vi "Get Shooter RPM.vi"() -> (1 "Average RPM":dbl, 2 "Right RPM":dbl, 3 "Left RPM":dbl)   [LabVIEW 2015]
uses:
  Robot Global Data.vi
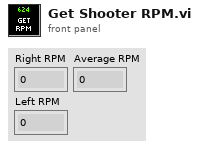
[diagram p1: front panel]
types:
  T1 = typedef "Dashboard Control Data.ctl" = cluster{"Auton Loops":dbl, "Shooter Presets":T2, "Encoder Control":T4, "Steer PID output":cluster{"output high":dbl, "output low":dbl}, " Steer PID gains":cluster{"proportional gain (Kc)":dbl, "integral time (Ti, min)":dbl, "derivative time (Td, min)":dbl}, "Drivetrain Settings":T5, "Vision Packet":T6, "Dashboard Drivetrain Command":T7}
  T2 = typedef "Shooter Presets.ctl" = cluster{"Batter Shot":T3, "Low Bar Curve Shot":T3, "Deep Middle Shot":T3, "Manual Shot":T3, "Left Ticks Per Rotation":dbl, "Right Ticks Per Rotation":dbl, "Low Bar Shot":T3, "Shooter RPM Tolerance":dbl, "IIR Filter Power":dbl}
  T3 = typedef "Shot Presets.ctl" = cluster{"Left Wheel RPM":dbl, "Right Wheel RPM":dbl}
  T4 = typedef "Encoder Control.ctl" = cluster{"Right Tick Constat":dbl, "Left Tick Constant":dbl, "Reset?":bool, "Y Dist":cluster{"PID gains":cluster{"proportional gain (Kc)":dbl, "integral time (Ti, min)":dbl, "derivative time (Td, min)":dbl}}, "Y Stop Thresh":dbl, "Y Stop Speed":dbl}
  T5 = typedef "Drivetrain Settings.ctl" = cluster{"Gyro Tolerance":dbl, "Throttle Ramp (ms)":dbl, "Angular rate compensation":bool, "Throttle to Rate Scale":dbl, "Rate compensation gain":dbl}
  T6 = typedef "Vision Packet.ctl" = cluster{"Distance":dbl, "Center X":dbl, "Center Y":dbl, "Found Target?":bool}
  T7 = typedef "Dashboard Drivetrain Command.ctl" = cluster{"Drivetrain Vision":T8, "Vision Scale Down Speed":dbl, "Vision PID gains":cluster{"proportional gain (Kc)":dbl, "integral time (Ti, min)":dbl, "derivative time (Td, min)":dbl}}
  T8 = typedef "Drivetrain Vision.ctl" = cluster{"High parameters":dbl, "Low parameters":dbl}
  T9 = typedef "WPI_EncoderDevRef.ctl" = cluster{"DevStatus":errorcluster, "EncoderIndex":T10, "CounterIndex":T11, "DistancePerCount":dbl, "Decoding Type":T12}
  T10 = typedef "FPGA_EncoderIdx.ctl" = enum8{"Enc 0", "Enc 1", "Enc 2", "Enc 3", "Enc 4", "Enc 5", "Enc 6", "Enc 7", "Invalid"}
  T11 = typedef "FPGA_CounterCtrSystemIndex.ctl" = enum8{"Ctr 0", "Ctr 1", "Ctr 2", "Ctr 3", "Ctr 4", "Ctr 5", "Ctr 6", "Ctr 7", "Invalid"}
  T12 = typedef "WPI_EncoderType.ctl" = enum16{"1x", "2x", "4x"}
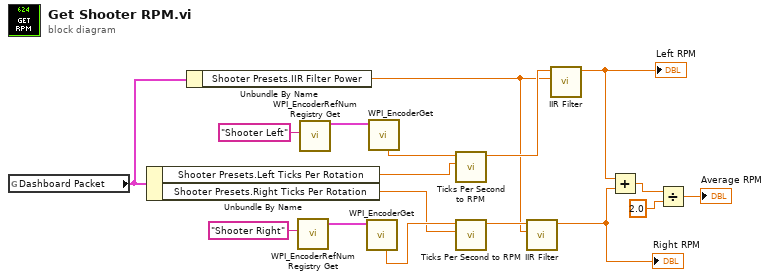
[diagram p0: block diagram]
diagram:
  n1 = global read "Robot Global Data.vi" "Dashboard Packet"() -> (w6:T1)
  n2 = Unbundle By Name(w6) -> ("Shooter Presets.Left Ticks Per Rotation"=w12:dbl, "Shooter Presets.Right Ticks Per Rotation"=w10:dbl)
  n3 = Unbundle By Name(w6) -> ("Shooter Presets.IIR Filter Power"=w1:dbl)
  n4 = call <vilib>:"WPI_EncoderRefNum Registry Get.vi"("refnum name"="Shooter Right") -> ("EncoderDevRef"=w14:T9)  [unwired: 9 in, 1 out]
  n5 = call <vilib>:"WPI_EncoderRefNum Registry Get.vi"("refnum name"="Shooter Left") -> ("EncoderDevRef"=w15:T9)  [unwired: 9 in, 1 out]
  n6 = call <vilib>:"WPI_EncoderGet.vi"("EncoderDevRef"=w14) -> ("Rate"=w11:dbl)  [unwired: 5 in, 5 out]
  n7 = call <vilib>:"WPI_EncoderGet.vi"("EncoderDevRef"=w15) -> ("Rate"=w13:dbl)  [unwired: 5 in, 5 out]
  n8 = call "Ticks Per Second to RPM.vi"("Ticks per Rotation"=w12, "Ticks Per Second"=w13) -> ("RPM"=w5:dbl)  [unwired: 9 in]
  n9 = call "Ticks Per Second to RPM.vi"("Ticks per Rotation"=w10, "Ticks Per Second"=w11) -> ("RPM"=w3:dbl)  [unwired: 9 in]
  n10 = call "IIR Filter.vi"("Filter Power"=w1, "Value"=w3) -> ("Filtered Value"=w2:dbl)  [unwired: 9 in]
  "Right RPM" <- w2
  n11 = call "IIR Filter.vi"("Filter Power"=w1, "Value"=w5) -> ("Filtered Value"=w4:dbl)  [unwired: 9 in]
  "Left RPM" <- w4
  n12 = Add(x=w4, y=w2) -> (x+y=w9:dbl)
  n13 = Divide(x=w9, y=2.0) -> (x/y=→"Average RPM":dbl)
